vi "Present.vi"(6 "Reverse Rows (T)":bool=TRUE, 11 "Pixel Data in":u32[][](array[numeric])) -> (3 "2D Picture":picture)   [LabVIEW 2022 SP3, in "Raster.lvlib"]
uses:
  Raster.lvlib
  <vilib>/Utility/High Resolution Relative Seconds.vi
  <vilib>/picture/picture.llb/Draw True-Color Pixmap.vi
  Utility/Utility.lvlib
panel:
  out "Present Time [s]":dbl format="%.1p"
  # "(0,0)"
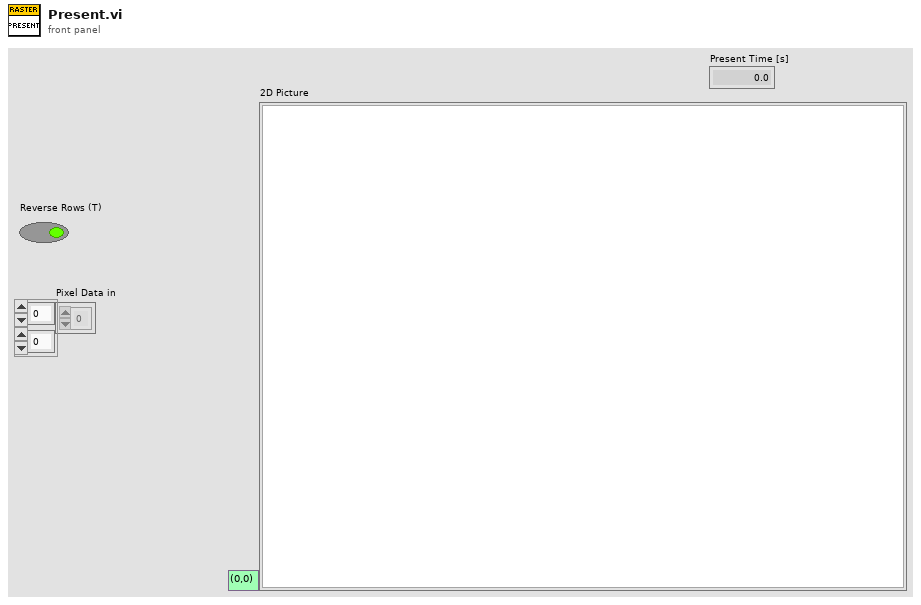
[diagram p1: front panel]
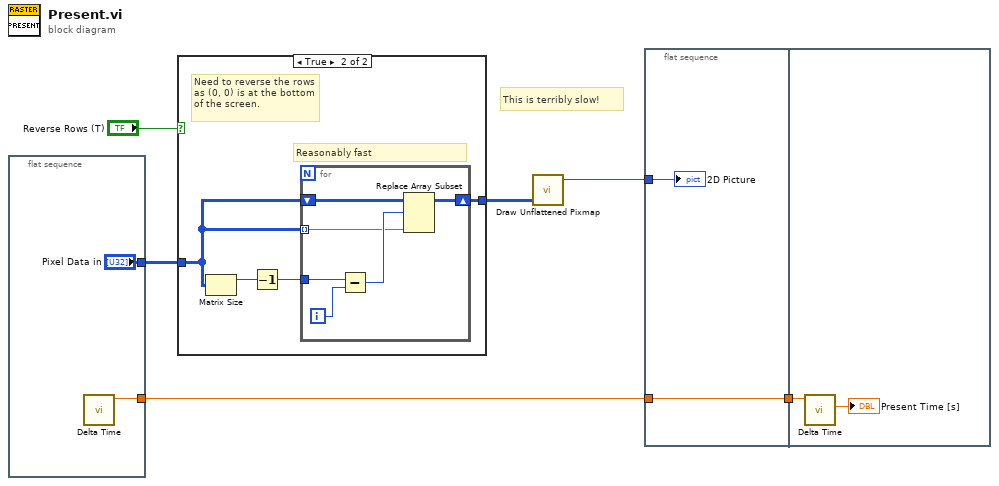
[diagram p0: block diagram]
diagram:
  # "This is terribly slow!"
  n1 = flat-sequence {
    tunnel: ["Pixel Data in"] -> w1
    tunnel: [w7] -> w3
    frame #0 {
      n2 = call "Delta Time.vi"() -> ("Relative Seconds Out"=w7:dbl)  [unwired: 10 in, 1 out]
    }
  }
  n3 = case shown="True" "Reverse Rows (T)" {
    tunnel: w1 -> [w9 w13]
    tunnel: [w9 w10] -> w4
    frame False {
    }
    frame True {
      # "Need to reverse the rows as (0, 0) is at the bottom of the screen."
      # "Reasonably fast"
      n4 = Matrix Size(0:w13) -> (1:w12:i32)  [unwired: 1 out]
      n5 = Decrement(x=w12) -> (x-1=w11:i32)
      n6 = for {
        tunnel: w13 -> [w15] mode=indexing
        shift-right: [w14] -> w10
        shift-left: w13 -> [w19]
        tunnel: w11 -> [w18]
        i -> [w17]
        n7 = Subtract(x=w18, y=w17) -> (x-y=w16:i32)
        n8 = Replace Array Subset(array=w19, new element=w15, index (row)=w16) -> (w14:u32[][])  [unwired: 1 in]
      }
    }
  }
  n9 = call-poly <vilib>:"Draw Unflattened Pixmap.vi"("data (RGB format)"=w4) -> ("new picture"=w6:picture)  [unwired: 8 in]
  n10 = flat-sequence {
    tunnel: w3 -> [w21]
    tunnel: w6 -> [w20]
    tunnel: [w21] -> w2
    tunnel: w2 -> [w23]
    frame #0 {
      "2D Picture" <- w20
    }
    frame #1 {
      n11 = call "Delta Time.vi"("Relative Seconds In"=w23) -> ("Delta Time [s]"=→"Present Time [s]":dbl)  [unwired: 9 in, 1 out]
    }
  }
